vi "centerHolo.vi"(6 "posCluster":T1={"1_Xoffset"=1329.0, "1_Yoffset"=-67.0, "1_Xgros"=0.04792332268370547, "1_Ygros"=-0.08130081300812986, "1_Xfine"=-1.2939297124600642, "1_Yfine"=0.18218623481781382, "1_Xreverse"=0, "1_Yreverse"=0, "1_XYswap"=0}, 7 "Ypos":dbl, 8 "Ycenter":dbl, 9 "Xpos":dbl, 10 "Xcenter":dbl) -> (1 "new Y gros":dbl, 3 "new X gros":dbl)   [LabVIEW 2023]
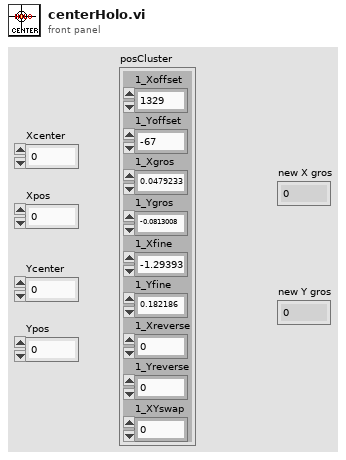
[diagram p1: front panel]
types:
  T1 = cluster{"1_Xoffset":dbl, "1_Yoffset":dbl, "1_Xgros":dbl, "1_Ygros":dbl, "1_Xfine":dbl, "1_Yfine":dbl, "1_Xreverse":u16, "1_Yreverse":u16, "1_XYswap":u16}
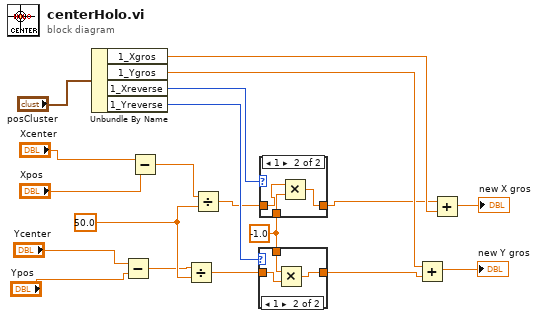
[diagram p0: block diagram]
diagram:
  w7 = -1.0
  w15 = 50.0 ("y")
  n1 = Unbundle By Name("posCluster") -> ("1_Xgros"=w3:dbl, "1_Ygros"=w4:dbl, "1_Xreverse"=w11:u16, "1_Yreverse"=w10:u16)
  n2 = Subtract(x="Ycenter", y="Ypos") -> (x-y=w14:dbl)
  n3 = Subtract(x="Xcenter", y="Xpos") -> (x-y=w13:dbl)
  n4 = Divide(x=w14, y=w15) -> (x/y=w8:dbl)
  n5 = Divide(x=w13, y=w15) -> (x/y=w9:dbl)
  n6 = case shown="1" w10 {
    tunnel: [w20 w21] -> w1
    tunnel: w8 -> [w20 w22]
    tunnel: w7 -> [_ w23]
    frame 0, Default {
    }
    frame 1 {
      n7 = Multiply(x=w23, y=w22) -> (x*y=w21:dbl)
    }
  }
  n8 = case shown="1" w11 {
    tunnel: [w24 w26] -> w2
    tunnel: w9 -> [w24 w25]
    tunnel: w7 -> [_ w27]
    frame 0, Default {
    }
    frame 1 {
      n9 = Multiply(x=w25, y=w27) -> (x*y=w26:dbl)
    }
  }
  n10 = Add(x=w4, y=w1) -> (x+y=→"new Y gros":dbl)
  n11 = Add(x=w2, y=w3) -> (x+y=→"new X gros":dbl)
